vi "LEP_RV_MemoryMap_Cmp.vi"(8 "error in (no error)":errorcluster, 10 "VI Config":T1, 11 "VI Path":path) -> (0 "error out":errorcluster, 3 "Match":bool)   [LabVIEW 2011]
doc: "Define the memory mapper compare operator for the Axiom CMD565 target."
uses:
  <vilib>/LabVIEW Targets/Embedded/Utilities/MemMap/EMB_Utility_MemMap_VI_Config.ctl
  <vilib>/LabVIEW Targets/Embedded/Utilities/MemMap/EMB_Utility_MemMap_VI_Type.ctl
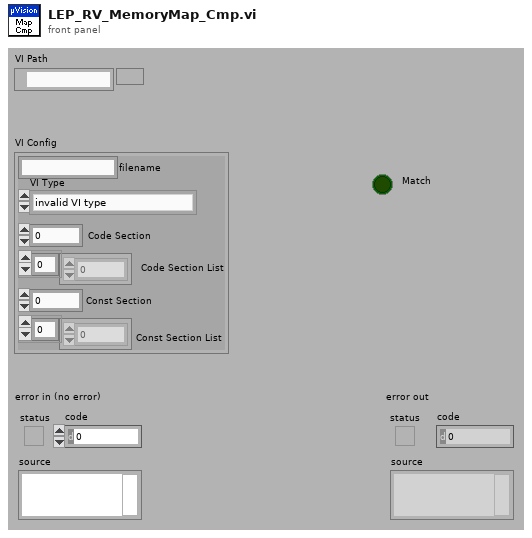
[diagram p1: front panel]
types:
  T1 = typedef "EMB_Utility_MemMap_VI_Config.ctl" = cluster{"filename":string, "Code Section":i32, "Code Section List":i32[], "Const Section":i32, "Const Section List":i32[], "VI Type":T2}
  T2 = typedef "EMB_Utility_MemMap_VI_Type.ctl" = enum32{"invalid VI type", "Standard VI", "Control VI", "Global VI", "Polymorphic VI", "Configuration VI", "SubSystem"}
  T3 = enum32{"invalid VI type", "Standard VI", "Control VI", "Global VI", "Polymorphic VI", "Configuration VI", "SubSystem", "Facade VI", "Method VI", "Statechart Diagram VI"}
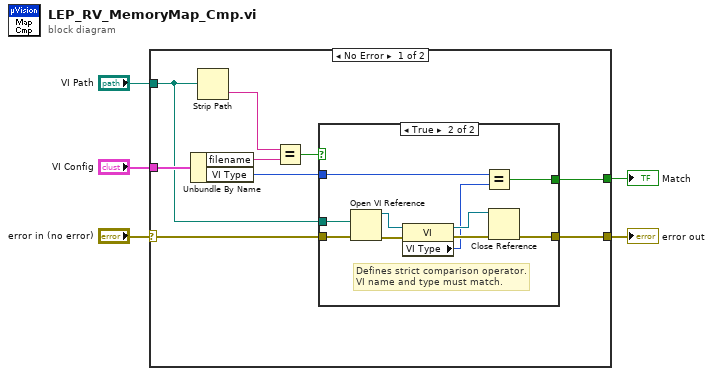
[diagram p0: block diagram]
diagram:
  n1 = case shown="No Error" "error in (no error)" {
    selector: "error in (no error)" -> [w11 w26]
    tunnel: [w10 w26] -> w4
    tunnel: "VI Config" -> [w14 _]
    tunnel: "VI Path" -> [w6 _]
    tunnel: [w8 _] -> w1
    frame No Error {
      n2 = Unbundle By Name(w14) -> ("filename"=w7:string, "VI Type"=w9:T2)
      n3 = Strip Path(path=w6) -> (name=w13:string)  [unwired: 1 out]
      n4 = Equal?(x=w13, y=w7) -> (x = y?=w12:bool)
      n5 = case shown="True" w12 {
        tunnel: w11 -> [w15 w25]
        tunnel: [w15 w20] -> w10
        tunnel: w9 -> [_ w19]
        tunnel: [_ w17] -> w8
        tunnel: w6 -> [_ w16]
        frame False {
        }
        frame True {
          # "Defines strict comparison operator. \nVI name and type must match."
          n6 = Open VI Reference(vi path=w16, error in (no error)=w25) -> (vi reference=w22:refnum<vi>, error out=w24:errorcluster)  [unwired: 4 in]
          n7 = property class="VI"(reference=w22, error in=w24) -> (reference out=w21:refnum<vi>, error out=w23:errorcluster, "VI Type"=w18:T3)
          n8 = Equal?(x=w19, y=w18) -> (x = y?=w17:bool)
          n9 = Close Reference(reference=w21, error in (no error)=w23) -> (error out=w20:errorcluster)
        }
      }
    }
    frame Error {
    }
  }
  "error out" <- w4
  "Match" <- w1
